vi "Acquire & Graph Continuous External Clock Sync.vi"() -> ()   [LabVIEW 8.6]
uses:
  vi.lib/UeiDaq/UeiDaqReadScaledData.vi
  vi.lib/UeiDaq/UeiDaqCreateAISession.vi
  vi.lib/UeiDaq/UeiDaqConfigureTimingForBufferedO.vi
  <libdir>/resource/objmgr/UeiDaq.rc
panel:
  in  "timeout (ms)":u32
  in  "range (V)":dbl
  in  "Analog Input Mode":enum16{"Differential", "Single-Ended"}(ring)
  out "Total scans acquired":u32[](array[numeric])
  in  "Resources":string[](array[string])
  out "Waveform Graph":dbl[][](graph)
  in  "Sampling rate":dbl
  in  "Number of samples  per channel":i32
  in  "stop":bool
  # "Resources names (master first if synchronization)"
  # "Analog input settings"
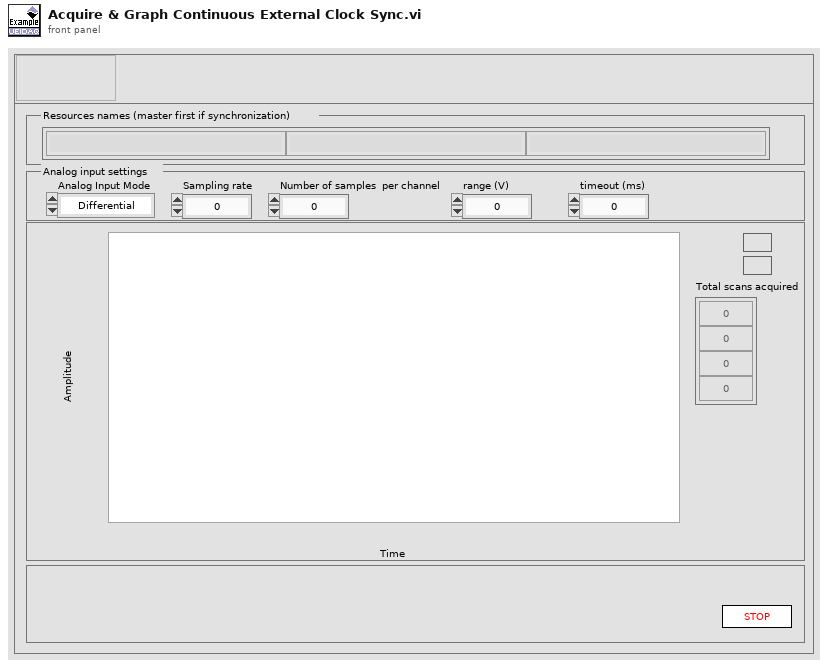
[diagram p1: front panel]
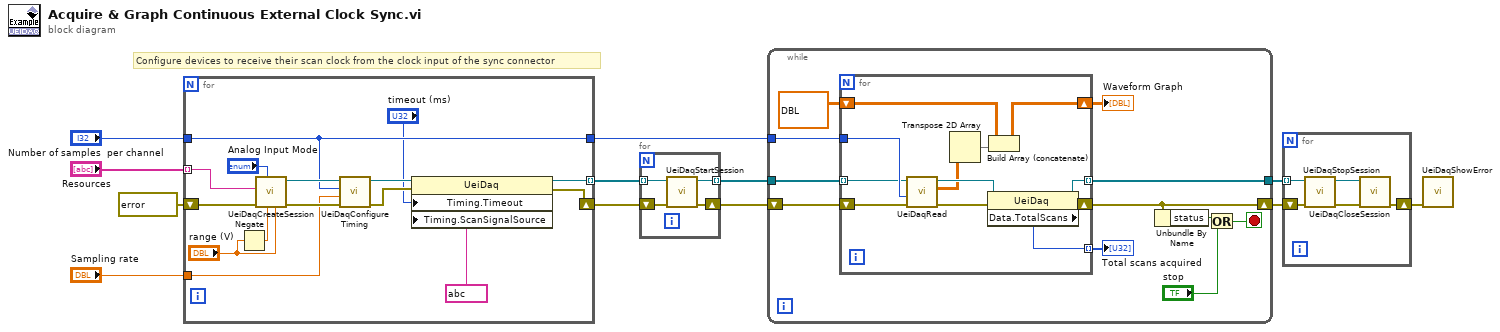
[diagram p0: block diagram]
diagram:
  # "Configure devices to receive their scan clock from the clock input of the sync connector"
  n1 = for {
    tunnel: [w23] -> w10
    tunnel: [w16] -> w2 mode=indexing
    shift-right: [w14] -> w7
    shift-left: errorcluster ? ("error out") -> [w25]
    tunnel: "Resources" -> [w24] mode=indexing
    tunnel: "Number of samples  per channel" -> [w23]
    tunnel: "Sampling rate" -> [w22]
    n2 = Negate(x="range (V)") -> (-x=w20:dbl)
    n3 = call-poly "UeiDaqCreateSession.vi"("Maximum range"="range (V)", "Minimum range"=w20, "Analog Input Mode"="Analog Input Mode", "error in (no error)"=w25, "Resource"=w24) -> ("error out"=w26:errorcluster, "UeiDaq Refnum Out"=w27:refnum<k20>)  [unwired: 1 in, 4 out]
    n4 = call-poly "UeiDaqConfigureTiming.vi"("error in (no error)"=w26, "Sampling rate"=w22, "Number of samples \nper channel"=w23, "UeiDaq Refnum In"=w27) -> ("error out"=w15:errorcluster, "UeiDaq Refnum Out"=w17:refnum<k20>)  [unwired: 3 in, 3 out]
    n5 = property class="UeiDaq"(reference=w17, error in=w15, "Timing.Timeout"="timeout (ms)", "Timing.ScanSignalSource"=string ?) -> (reference out=w16:refnum<k20>, error out=w14:errorcluster)
  }
  n6 = for {
    tunnel: [w31] -> w1 mode=indexing
    tunnel: w2 -> [w28] mode=indexing
    shift-right: [w30] -> w11
    shift-left: w7 -> [w29]
    n7 = call "UeiDaqStartSession.vi"("error in (no error)"=w29, "UeiDaq Refnum In"=w28) -> ("error out"=w30:errorcluster, "UeiDaq Refnum Out"=w31:refnum<k20>)  [unwired: 8 out]
  }
  n8 = while {
    tunnel: w1 -> [w37]
    tunnel: [w36] -> w9
    tunnel: w10 -> [w38]
    shift-right: [w32] -> w8
    shift-left: w11 -> [w39]
    stop <- w40 stop-if-true
    n9 = for {
      tunnel: w38 -> [w53]
      tunnel: w37 -> [w52] mode=indexing
      tunnel: [w51] -> w36 mode=indexing
      shift-right: [w48] -> w32
      shift-left: w39 -> [w54]
      tunnel: [w47] -> w35 mode=indexing
      shift-right: [w45] -> w33
      shift-left: dbl[][] ? -> [w44]
      n10 = call-poly "UeiDaqRead.vi"("error in (no error)"=w54, "numScans"=w53, "UeiDaq Refnum In"=w52) -> ("error out"=w49:errorcluster, "Scaled Data"=w46:dbl[][], "UeiDaq Refnum Out"=w50:refnum<k20>)  [unwired: 6 out]
      n11 = Transpose 2D Array(2D array=w46) -> (transposed array=w43:dbl[][])
      n12 = property class="UeiDaq"(reference=w50, error in=w49) -> (reference out=w51:refnum<k20>, error out=w48:errorcluster, "Data.TotalScans"=w47:u32)
      n13 = Build Array (concatenate)(w44, w43) -> (w45:dbl[][])
    }
    "Waveform Graph" <- w33
    "Total scans acquired" <- w35
    n14 = Unbundle By Name(w32) -> ("status"=w42:bool)
    n15 = Or(x=w42, y="stop") -> (x .or. y?=w40:bool)
  }
  n16 = for {
    tunnel: w9 -> [w58] mode=indexing
    shift-right: [w59] -> w12
    shift-left: w8 -> [w56]
    n17 = call "UeiDaqStopSession.vi"("error in (no error)"=w56, "UeiDaq Refnum In"=w58) -> ("error out"=w55:errorcluster, "UeiDaq Refnum Out"=w57:refnum<k20>)  [unwired: 8 out]
    n18 = call "UeiDaqCloseSession.vi"("error in (no error)"=w55, "UeiDaq Refnum In"=w57) -> ("error out"=w59:errorcluster)  [unwired: 1 in, 8 out]
  }
  n19 = call "UeiDaqShowError.vi"("error in (no error)"=w12) -> ()  [unwired: 1 in, 10 out]
